vi "smooth 130415.vi"(1 "window size":i32, 2 "dimension size":i32, 3 "initialized array":i32[](array[numeric]), 4 "Array":i16[](array[numeric])=[0, 0, 0, 0]) -> (0 "Array 2":i32[](array[numeric]))   [LabVIEW 2009]
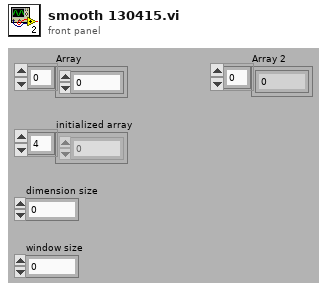
[diagram p1: front panel]
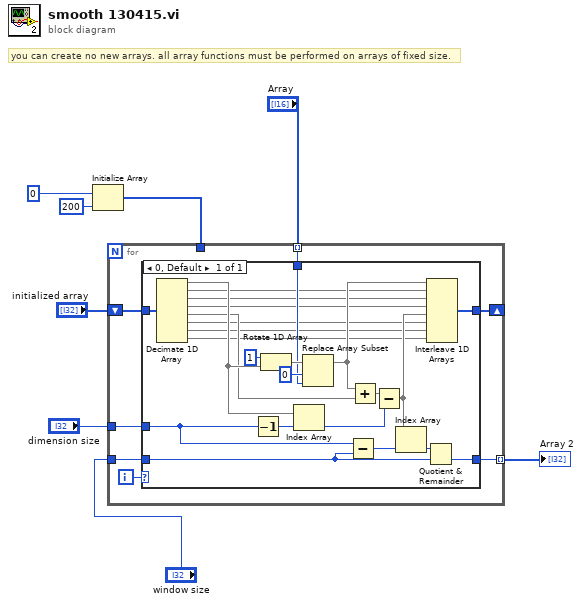
[diagram p0: block diagram]
diagram:
  # "you can create no new arrays. all array functions must be performed on arrays of fixed size."
  n1 = Initialize Array(0 ("dimension size"), 200 ("dimension size")) -> (w1:i32[])
  n2 = for {
    tunnel: "dimension size" -> [w14]
    tunnel: [w13] -> w7 mode=indexing
    tunnel: "window size" -> [w12]
    tunnel: "Array" -> [w10] mode=indexing
    shift-right: [w15] -> _
    shift-left: "initialized array" -> [w9]
    tunnel: w1 -> [_]
    i -> [w11]
    n3 = case shown="0, Default" w11 {
      tunnel: [w27] -> w15
      tunnel: w9 -> [w29]
      tunnel: w14 -> [w25]
      tunnel: [w22] -> w13
      tunnel: w12 -> [w23]
      tunnel: w10 -> [w26]
      frame 0, Default {
        n4 = Decimate 1D Array(w29) -> (w32:i32[], w21:i32[], w20:i32[], w19:i32[], w31:i32[], w18:i32[], w17:i32[], w16:i32[])
        n5 = Decrement(x=w25) -> (x-1=w36:i32)
        n6 = Rotate 1D Array(1:w32, 2:1 ("n")) -> (0:w38:i32[])
        n7 = Index Array(array=w32, index=w36) -> (element=w35:i32)
        n8 = Replace Array Subset(array=w38, new element=w26, index=0 ("n")) -> (w30:i32[])
        n9 = Subtract(x=w25, y=w23) -> (x-y=w33:i32)
        n10 = Add(x=w30, y=w31) -> (x+y=w34:i32[])
        n11 = Subtract(x=w34, y=w35) -> (x-y=w28:i32[])
        n12 = Index Array(array=w28, index=w33) -> (element=w24:i32)
        n13 = Quotient & Remainder(x=w24, y=w23) -> (floor(x/y)=w22:i32)  [unwired: 1 out]
        n14 = Interleave 1D Arrays(w30, w21, w20, w19, w28, w18, w17, w16) -> (w27:i32[])
      }
    }
  }
  "Array 2" <- w7
